vi "Follow Trajectory.vi"(1 "Time After Done[sec]":dbl, 2 "Drive Name":string="Drive", 3 "Motion Profile":T1(array[cluster])) -> ()   [LabVIEW 2016]
uses:
  <vilib>/Rock Robotics/WPI/Utilities/WPI_GetSetVariantRefNum.vi
  <vilib>/addons/control/pid/pid.llb/PID Control Input Filter (DBL).vi
  <vilib>/Rock Robotics/WPI/RobotDrive/WPI_RobotDriveArcadeDrive_Standard(NoSaturation).vi
  <vilib>/addons/control/pid/NI_PID_pid.lvlib
panel:
  out "dt":u32
  out "V Right":dbl
  out "V Left":dbl
  out "Distance L":dbl
  out "Distance R":dbl
  out "Robot Position":cluster{dbl[], dbl[]}[](graph)
  out "Angle Error":dbl(graph)
  in  "Kv":dbl=0.008
  in  "Ka":dbl
  out "element":T2
  in  "Drive PID Gains":cluster{"Kp":dbl, "Ki":dbl, "Kd":dbl}={"Kp"=-0.1, "Ki"=0.0, "Kd"=0.0}
  in  "Angle PID Gains":cluster{"Kp":dbl, "Ki":dbl, "Kd":dbl}={"Kp"=0.03, "Ki"=0.0, "Kd"=0.005}
  out "Distance* Error":dbl(graph)
  out "Total Time":dbl
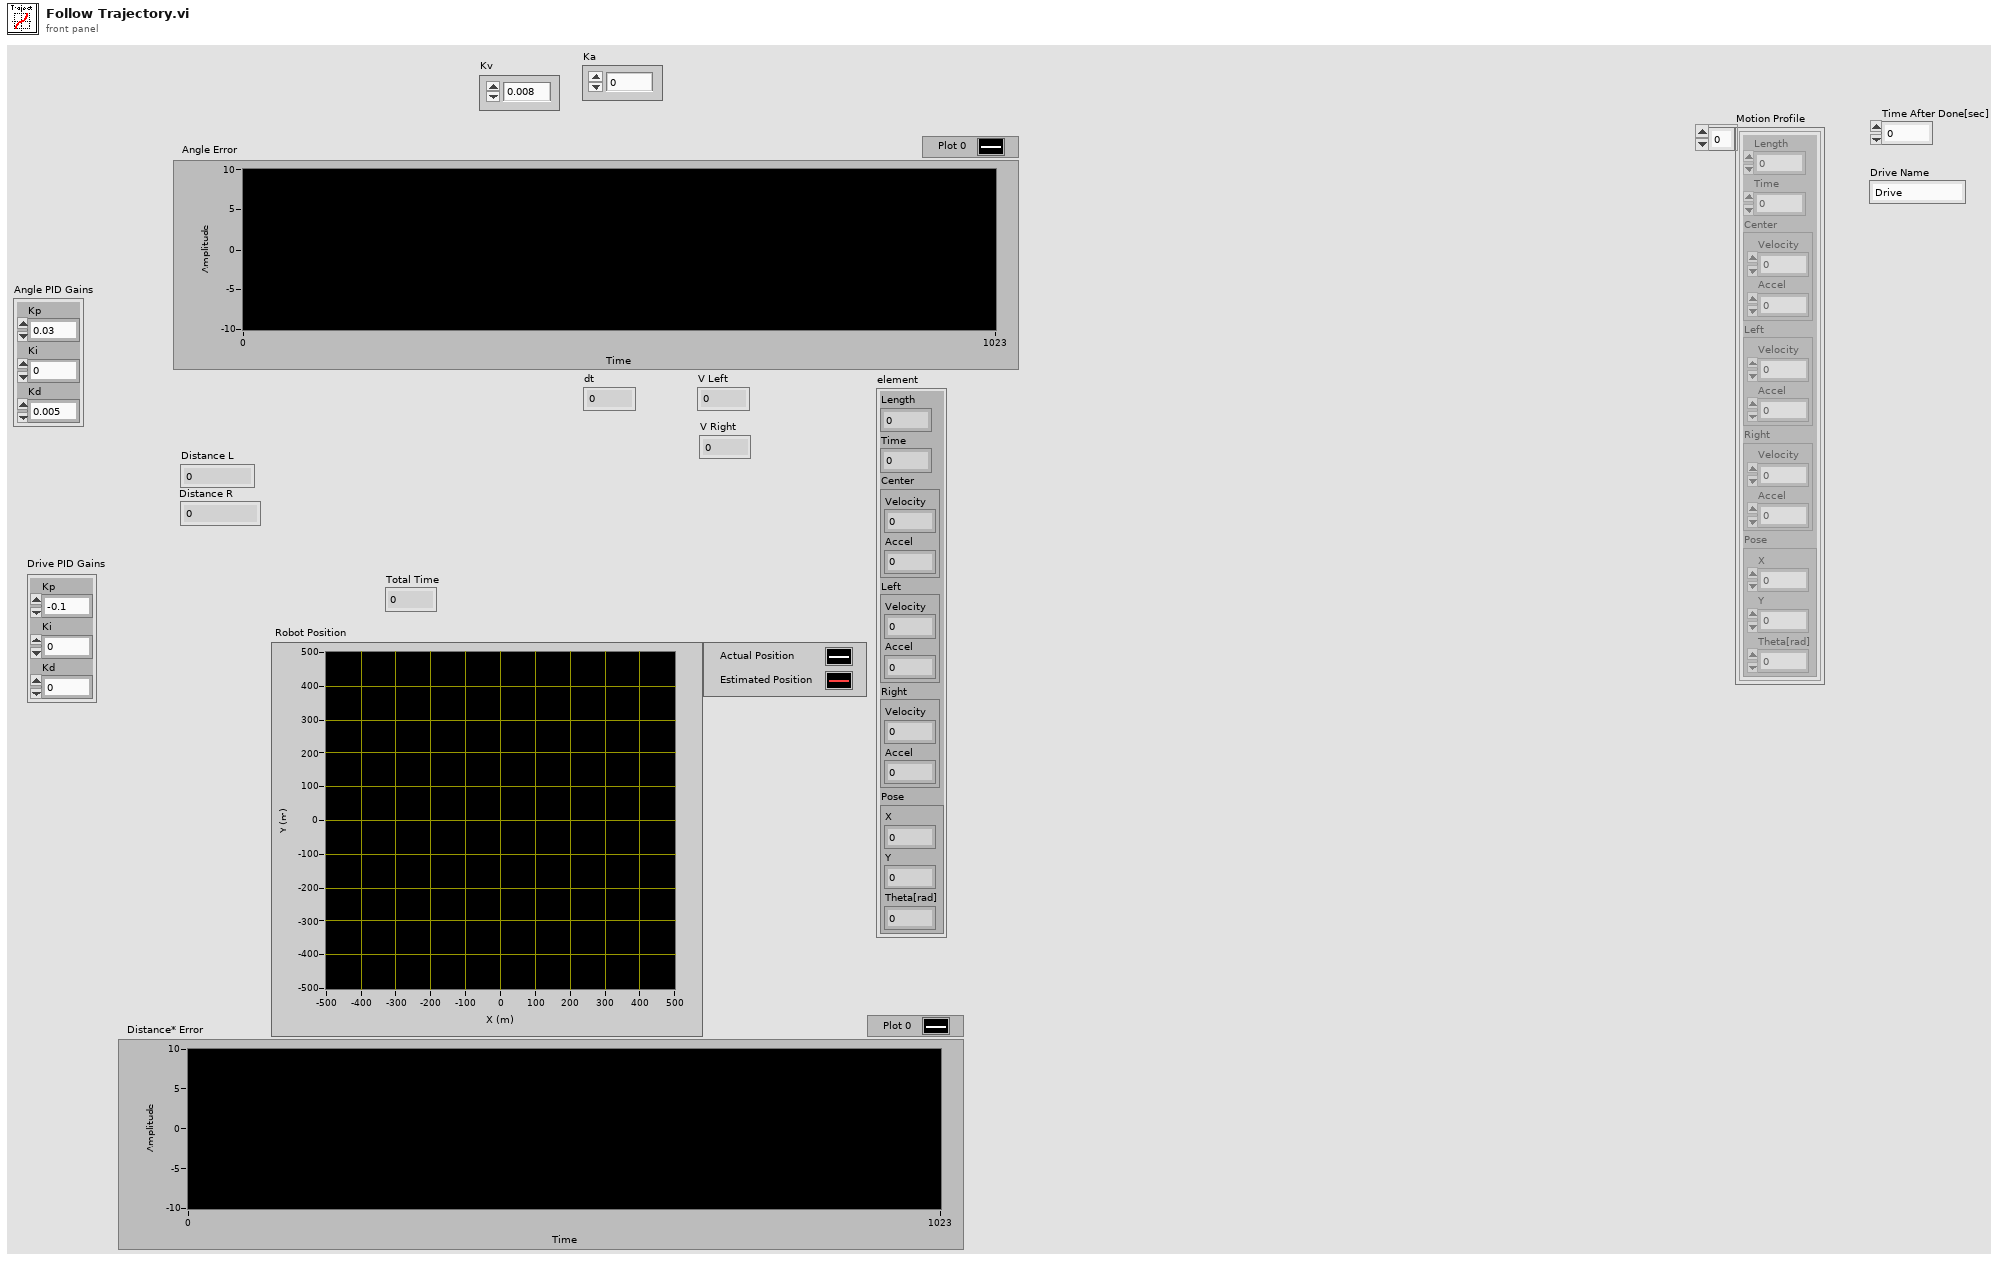
[diagram p1: front panel]
types:
  T1 = cluster{"Length":dbl, "Time":dbl, "Center":cluster{"Velocity":dbl, "Accel":dbl}, "Left":cluster{"Velocity":dbl, "Accel":dbl}, "Right":cluster{"Velocity":dbl, "Accel":dbl}, "Pose":cluster{"X":dbl, "Y":dbl, "Theta[rad]":dbl}}[]
  T2 = cluster{"Length":dbl, "Time":dbl, "Center":cluster{"Velocity":dbl, "Accel":dbl}, "Left":cluster{"Velocity":dbl, "Accel":dbl}, "Right":cluster{"Velocity":dbl, "Accel":dbl}, "Pose":cluster{"X":dbl, "Y":dbl, "Theta[rad]":dbl}}
  T3 = typedef "WPI_EncoderDevRef.ctl" = cluster{"DevStatus":errorcluster, "EncoderIndex":T4, "CounterIndex":T5, "DistancePerCount":dbl, "Decoding Type":T6}
  T4 = typedef "FPGA_EncoderIdx.ctl" = enum8{"Enc 0", "Enc 1", "Enc 2", "Enc 3", "Enc 4", "Enc 5", "Enc 6", "Enc 7", "Invalid"}
  T5 = typedef "FPGA_CounterCtrSystemIndex.ctl" = enum8{"Ctr 0", "Ctr 1", "Ctr 2", "Ctr 3", "Ctr 4", "Ctr 5", "Ctr 6", "Ctr 7", "Invalid"}
  T6 = typedef "WPI_EncoderType.ctl" = enum16{"1x", "2x", "4x"}
  T7 = cluster{"Yaw":dbl, "Roll":dbl, "Pitch":dbl, "Heading":dbl, "Fused Heading":dbl}
  T8 = typedef "WPI_RobotDriveDevRef.ctl" = cluster{"DevStatus":errorcluster, "Motors[]":T9[], "Square Inputs":bool, "Max Output":dbl}
  T9 = typedef "WPI_MotorControlDeviceRef.ctl" = cluster{"DeviceStatus":errorcluster, "Type":T10, "PWM":cluster{"PWM Channel":T11, "DeadBand":T12}, "CAN":cluster{"Device Number":u8, "SetOutput VI Ref":variant, "GetOutput VI Ref":variant, "Enable VI Ref":variant, "Disable VI Ref":variant, "Data":variant}, "Invert":bool}
  T10 = typedef "WPI_MotorControlType.ctl" = enum16{"PWM", "CAN"}
  T11 = typedef "FPGA_DIOPWMChannel.ctl" = enum8{"PWM 0", "PWM 1", "PWM 2", "PWM 3", "PWM 4", "PWM 5", "PWM 6", "PWM 7", "PWM 8", "PWM 9", "PWM MXP 0", "PWM MXP 1", "PWM MXP 2", "PWM MXP 3", "PWM MXP 4", "PWM MXP 5", "PWM MXP 6", "PWM MXP 7", "PWM MXP 8", "PWM MXP 9", "Invalid"}
  T12 = typedef "WPI_PWMDeadband.ctl" = cluster{"Name":string, "maxPositivePwm":i32, "minPositivePwm":i32, "centerPwm":i32, "maxNegativePwm":i32, "minNegativePwm":i32, "angularRange":u16}
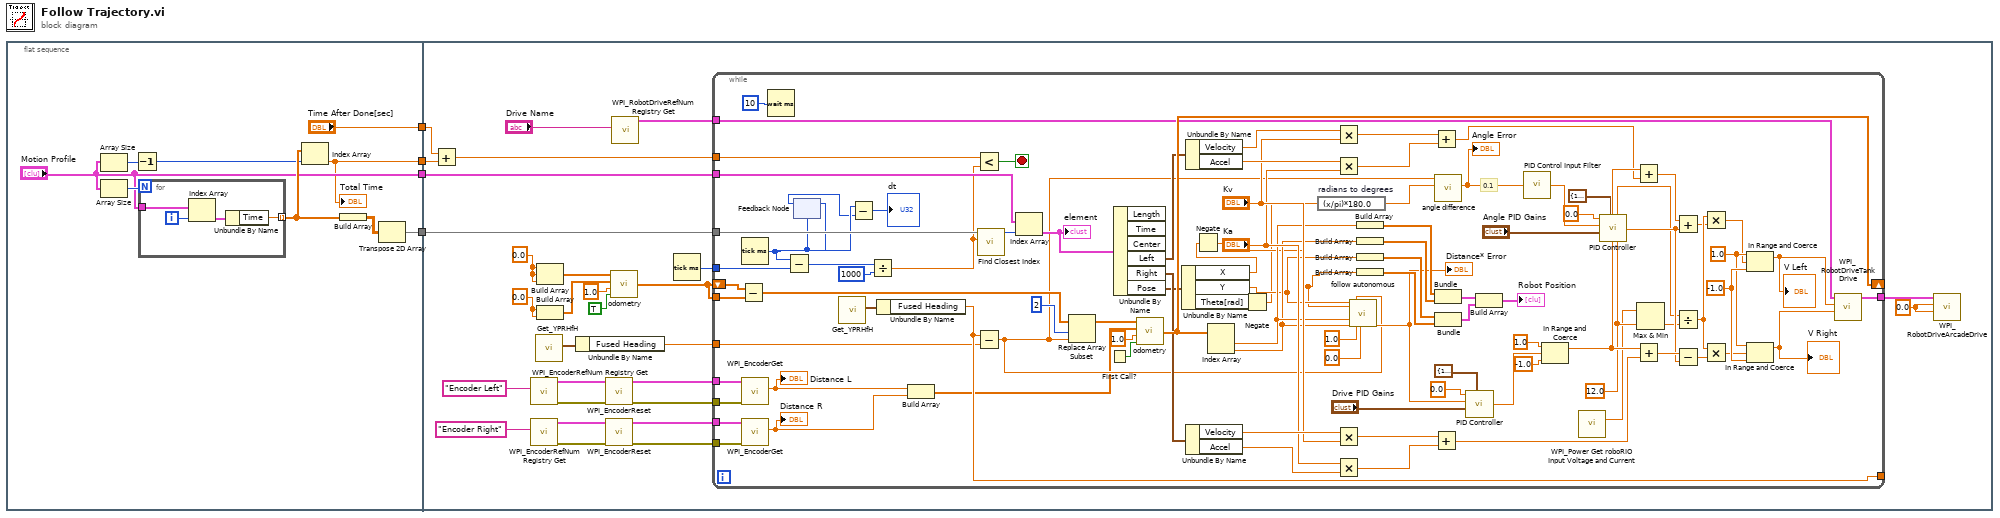
[diagram p0: block diagram]
diagram:
  n1 = flat-sequence {
    tunnel: [w11] -> w4
    tunnel: ["Motion Profile"] -> w3
    tunnel: [w6] -> w2
    tunnel: ["Time After Done[sec]"] -> w1
    tunnel: w4 -> [w39]
    tunnel: w3 -> [w38]
    tunnel: w2 -> [w36]
    tunnel: w1 -> [w37]
    frame #0 {
      n2 = Array Size(array="Motion Profile") -> (size(s)=w7:i32)
      n3 = Array Size(array="Motion Profile") -> (size(s)=w13:i32)
      n4 = Decrement(x=w7) -> (x-1=w8:i32)
      n5 = for {
        N: w13 -> [_]
        tunnel: "Motion Profile" -> [w17]
        tunnel: [w14] -> w10 mode=indexing
        i -> [w16]
        n6 = Index Array(array=w17, index=w16) -> (element=w15:T2)
        n7 = Unbundle By Name(w15) -> ("Time"=w14:dbl)
      }
      n8 = Index Array(array=w10, index=w8) -> (element=w6:dbl)
      "Total Time" <- w6
      n9 = Build Array(w10) -> (w12:dbl[][])
      n10 = Transpose 2D Array(2D array=w12) -> (transposed array=w11:dbl[][])
    }
    frame #1 {
      w44 = 0.0 ("element")
      w45 = 0.0 ("element")
      w29 = 0.0 ("Y axis value")
      n11 = Add(x=w37, y=w36) -> (x+y=w35:dbl)
      n12 = call <vilib>:"WPI_EncoderRefNum Registry Get.vi"("refnum name"="Encoder Left") -> ("error out"=w24:errorcluster, "EncoderDevRef"=w25:T3)  [unwired: 9 in]
      n13 = call <vilib>:"WPI_EncoderRefNum Registry Get.vi"("refnum name"="Encoder Right") -> ("error out"=w20:errorcluster, "EncoderDevRef"=w21:T3)  [unwired: 9 in]
      n14 = call <vilib>:"Get_YPRHfH.vi"() -> ("YRPHfH"=w32:T7)  [unwired: 11 in]
      n15 = Build Array(w45, w45, w45) -> (w40:dbl[])
      n16 = Build Array(w44, w44) -> (w43:dbl[])
      n17 = Unbundle By Name(w32) -> ("Fused Heading"=w33:dbl)
      n18 = call <vilib>:"WPI_EncoderReset.vi"("error in (no error)"=w24, "EncoderDevRef"=w25) -> ("error out"=w22:errorcluster, "EncoderDevRef"=w23:T3)  [unwired: 8 in]
      n19 = call <vilib>:"WPI_EncoderReset.vi"("error in (no error)"=w20, "EncoderDevRef"=w21) -> ("error out"=w18:errorcluster, "EncoderDevRef"=w19:T3)  [unwired: 8 in]
      n20 = call "odometry.vi"("reset"=TRUE, "distance between sides of wheels"=1.0, "encoders in"=w43, "state in"=w40) -> ("state out"=w34:dbl[])
      n21 = call <vilib>:"WPI_RobotDriveRefNum Registry Get.vi"("refnum name"="Drive Name") -> ("RobotDriveDevRef"=w30:T8)  [unwired: 9 in, 1 out]
      n22 = Tick Count (ms)() -> (millisecond timer value=w46:u32)
      n23 = while {
        tunnel: w46 -> [w140]
        tunnel: w30 -> [w67]
        tunnel: [w68] -> w28
        shift-right: [w126] -> _
        shift-left: w34 -> [w86]
        tunnel: w23 -> [w64]
        tunnel: w22 -> [w63]
        tunnel: w19 -> [w61]
        tunnel: w18 -> [w60]
        tunnel: [w80] -> _
        tunnel: w39 -> [w120]
        tunnel: w38 -> [w118]
        tunnel: w34 -> [w85]
        tunnel: w35 -> [w83]
        tunnel: w33 -> [w79]
        stop <- w81 stop-if-true
        w75 = 12.0 ("y")
        w125 = -1.0 ("lower limit")
        w124 = 1.0 ("upper limit")
        # "0.1"
        n24 = Subtract(x=w86, y=w85) -> (x-y=w84:dbl[])
        n25 = Tick Count (ms)() -> (millisecond timer value=w54:u32)
        n26 = call <vilib>:"WPI_EncoderGet.vi"("error in (no error)"=w63, "EncoderDevRef"=w64) -> ("Distance"=w62:dbl)  [unwired: 4 in, 5 out]
        "Distance L" <- w62
        n27 = call <vilib>:"WPI_EncoderGet.vi"("error in (no error)"=w60, "EncoderDevRef"=w61) -> ("Distance"=w59:dbl)  [unwired: 4 in, 5 out]
        "Distance R" <- w59
        n28 = Wait (ms)(milliseconds to wait=u32 10) -> ()  [unwired: 1 out]
        n29 = Subtract(x=w54, y=w140) -> (x-y=w101:u32)
        n30 = feedback-in #1(w54) -> ()
        n31 = feedback #1(w54) -> (w53:u32)
        n32 = call <vilib>:"Get_YPRHfH.vi"() -> ("YRPHfH"=w76:T7)  [unwired: 11 in]
        n33 = Subtract(x=w54, y=w53) -> (x-y=→"dt":u32)
        n34 = Divide(x=w101, y=u32 1000) -> (x/y=w82:dbl)
        n35 = Unbundle By Name(w76) -> ("Fused Heading"=w80:dbl)
        n36 = Build Array(w62, w59) -> (w51:dbl[])
        n37 = Less?(x=w83, y=w82) -> (x < y?=w81:bool)
        n38 = Subtract(x=w80, y=w79) -> (x-y=w77:dbl)
        n39 = call "Find Closest Index.vi"("Time"=w82, "Array"=w120) -> ("Index"=w119:i32)  [unwired: 9 in]
        n40 = Index Array(array=w118, index=w119) -> (element=w117:T2)
        "element" <- w117
        n41 = Replace Array Subset(array=w84, new element=w77, index=2) -> (w134:dbl[])
        n42 = First Call?() -> (First Call?: T/F=w131:bool)
        n43 = Unbundle By Name(w117) -> ("Left"=w116:cluster{"Velocity":dbl, "Accel":dbl}, "Right"=w115:cluster{"Velocity":dbl, "Accel":dbl}, "Pose"=w104:cluster{"X":dbl, "Y":dbl, "Theta[rad]":dbl})  [unwired: 3 out]
        n44 = call "odometry.vi"("reset"=w131, "distance between sides of wheels"=1.0, "encoders in"=w51, "state in"=w134) -> ("state out"=w126:dbl[])
        n45 = Unbundle By Name(w104) -> ("X"=w49:dbl, "Y"=w50:dbl, "Theta[rad]"=w103:dbl)
        n46 = Unbundle By Name(w116) -> ("Velocity"=w114:dbl, "Accel"=w113:dbl)
        n47 = Unbundle By Name(w115) -> ("Velocity"=w108:dbl, "Accel"=w105:dbl)
        n48 = Negate(x=w49) -> (-x=w48:dbl)
        n49 = Index Array(array=w126) -> (element #1=w99:dbl, element #2=w78:dbl)  [unwired: 2 in]
        n50 = Negate(x=w103) -> (-x=w47:dbl)
        n51 = expression code="(x/pi)*180.0" "radians to degrees"(w47) -> (w102:dbl)
        n52 = Multiply(x=w114, y="Kv") -> (x*y=w111:dbl)
        n53 = Multiply(x=w113, y="Ka") -> (x*y=w112:dbl)
        n54 = Multiply(x=w108, y="Kv") -> (x*y=w110:dbl)
        n55 = Multiply(x="Ka", y=w105) -> (x*y=w109:dbl)
        n56 = call "follow autonomous.vi"("x"=w50, "y"=w48, "robot x"=w99, "robot y"=w78, "robot angle"=w77, "speed kp"=1.0, "v"=0.0) -> ("newV"=w87:dbl)  [unwired: 12 in]
        "Distance* Error" <- w87
        n57 = Build Array(w99) -> (w137:dbl[])
        n58 = Build Array(w78) -> (w138:dbl[])
        n59 = Build Array(w50) -> (w123:dbl[])
        n60 = Build Array(w48) -> (w122:dbl[])
        n61 = Add(x=w111, y=w112) -> (x+y=w56:dbl)
        n62 = Add(x=w110, y=w109) -> (x+y=w55:dbl)
        n63 = call "angle difference.vi"("angle2"=w102, "angle1"=w77) -> ("angle diff"=w89:dbl)  [unwired: 9 in]
        "Angle Error" <- w89
        n64 = Bundle(w137, w138) -> (w136:cluster{dbl[], dbl[]})  [unwired: 1 in]
        n65 = Bundle(w123, w122) -> (w121:cluster{dbl[], dbl[]})  [unwired: 1 in]
        n66 = call "PID Controller.vi"("setpoint"=0.0, "process variable"=w87, "PID Gains"="Drive PID Gains", "Constrain"=cluster{"Max Control":dbl, "Min Control":dbl} {"Max Control"=1.0, "Min Control"=-1.0}) -> ("Control Signal"=w90:dbl)  [unwired: 1 in]
        n67 = Build Array(w136, w121) -> (→"Robot Position":cluster{dbl[], dbl[]}[])
        n68 = call-poly <vilib>:"PID Control Input Filter.vi"("input"=w89) -> ("output"=w88:dbl)  [unwired: 4 in]
        n69 = In Range and Coerce(upper limit=1.0, x=w90, lower limit=-1.0) -> (coerced(x)=w129:dbl)  [unwired: 1 out]
        n70 = call <vilib>:"WPI_Power Get roboRIO Input Voltage and Current.vi"() -> ("roboRIO input voltage (V)"=w74:dbl)  [unwired: 13 in, 2 out]
        n71 = call "PID Controller.vi"("setpoint"=0.0, "process variable"=w88, "PID Gains"="Angle PID Gains", "Constrain"=cluster{"Max Control":dbl, "Min Control":dbl} {"Max Control"=1.0, "Min Control"=-1.0}) -> ("Control Signal"=w92:dbl)  [unwired: 1 in]
        n72 = Add(x=w129, y=w56) -> (x+y=w69:dbl)
        n73 = Add(x=w129, y=w55) -> (x+y=w130:dbl)
        n74 = Max & Min(x=w74, y=w75) -> (min(x,y)=w73:dbl)  [unwired: 1 out]
        n75 = Add(x=w69, y=w92) -> (x+y=w58:dbl)
        n76 = Divide(x=w75, y=w73) -> (x/y=w70:dbl)
        n77 = Subtract(x=w130, y=w92) -> (x-y=w57:dbl)
        n78 = Multiply(x=w70, y=w58) -> (x*y=w72:dbl)
        n79 = Multiply(x=w70, y=w57) -> (x*y=w71:dbl)
        n80 = In Range and Coerce(upper limit=w124, x=w72, lower limit=w125) -> (coerced(x)=w65:dbl)  [unwired: 1 out]
        "V Left" <- w65
        n81 = In Range and Coerce(upper limit=w124, x=w71, lower limit=w125) -> (coerced(x)=w66:dbl)  [unwired: 1 out]
        "V Right" <- w66
        n82 = call <vilib>:"WPI_RobotDriveTankDrive.vi"("Right axis value"=w66, "Left axis value"=w65, "RobotDriveDevRef"=w67) -> ("RobotDriveDevRef"=w68:T8)  [unwired: 6 in, 2 out]
      }
      n83 = call-poly <vilib>:"WPI_RobotDriveArcadeDrive.vi"("Y axis value"=w29, "X axis value"=w29, "RobotDriveDevRef"=w28) -> ()  [unwired: 6 in, 3 out]
    }
  }
